vi "local varibales 2.vi"() -> ()   [LabVIEW 2024]
panel:
  out "Numeric 3":dbl
  out "Numeric 2":dbl
  out "x^y 2":dbl
  out "x^y":dbl
  in  "Numeric":dbl
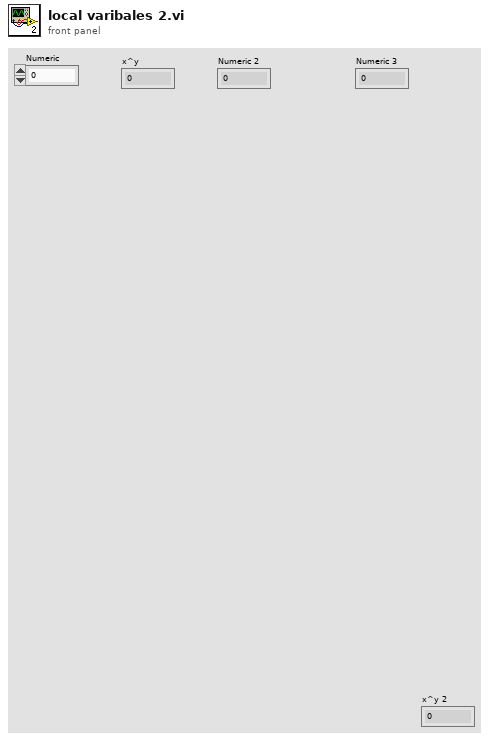
[diagram p1: front panel]
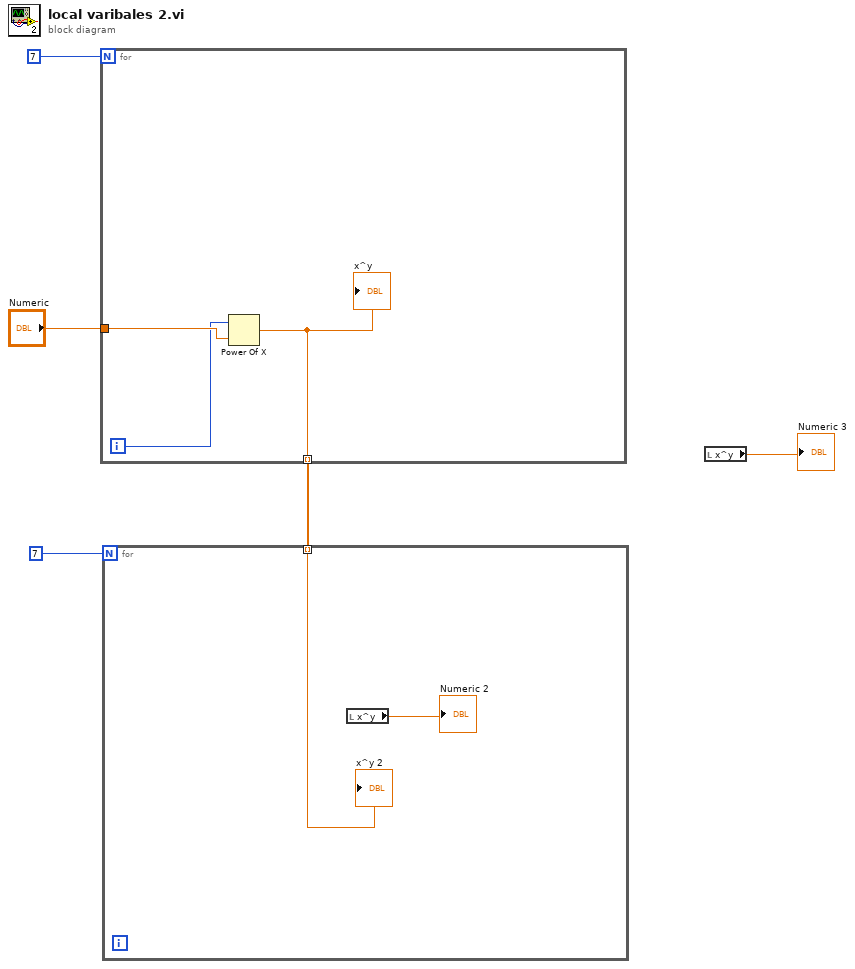
[diagram p0: block diagram]
diagram:
  n1 = for {
    N: 7 -> [_]
    tunnel: "Numeric" -> [w8]
    tunnel: [w6] -> w2 mode=indexing
    i -> [w7]
    n2 = Power Of X(1:w8, 2:w7) -> (0:w6:dbl)
    "x^y" <- w6
  }
  n3 = for {
    N: 7 -> [_]
    tunnel: w2 -> [w10] mode=indexing
    n4 = local read "x^y"() -> (→"Numeric 2":dbl)
    "x^y 2" <- w10
  }
  n5 = local read "x^y"() -> (→"Numeric 3":dbl)
